vi "Determine Steps.vi"(8 "error in (no error)":errorcluster, 11 "DataProcessor in":refnum<class "DataProcessor.lvclass">) -> (0 "error out":errorcluster, 3 "DataProcessor out":refnum<class "DataProcessor.lvclass">)   [LabVIEW 2020, in "Volatus.lvlib" / "DataProcessor.lvclass"]
uses:
  DataProcessor.lvclass
  DataProcessor.lvclass/DataProcessor.ctl
  Task/Task.lvclass
  VolatusConfig/VolatusConfigElement/VolatusConfigElement.lvclass
  Processing Type.ctl
  Volatus.lvlib
  VolatusConfig/Task/Task.lvclass
  C:/dev/lv20CE/relink/lv-volatus/VolatusConfig/VolatusConfigElement/VolatusConfigElement.lvclass
  C:/dev/lv20CE/relink/lv-volatus/VolatusConfig/Task/Task.lvclass
  C:/dev/lv20CE/relink/lv-volatus/Volatus/DataHandlerTask/DataHandlerTask.lvclass
  C:/dev/lv20CE/relink/lv-volatus/Volatus/Task/Task.lvclass
  C:/Program Files (x86)/National Instruments/LabVIEW 2020/vi.lib/ActorFramework/Actor/Actor.lvclass
  C:/dev/lv20CE/relink/lv-volatus/Volatus/TaskStateHandler/TaskStateHandler.lvclass
  C:/dev/lv20CE/relink/lv-volatus/Volatus/VectoMessageHandler/VectoMessageHandler.lvclass
  C:/dev/lv20CE/relink/lv-volatus/Volatus/API Provider/API Provider.lvclass
  C:/dev/lv20CE/relink/lv-volatus/Volatus/DataHandler/DataHandler.lvclass
  C:/dev/lv20CE/relink/lv-volatus/Volatus/DataProcessor/DataProcessor.lvclass
  C:/dev/lv20CE/relink/lv-volatus/Volatus/Abortable/Abortable.lvclass
  C:/dev/lv20CE/relink/lv-volatus/Volatus/Reconfigurable/Reconfigurable.lvclass
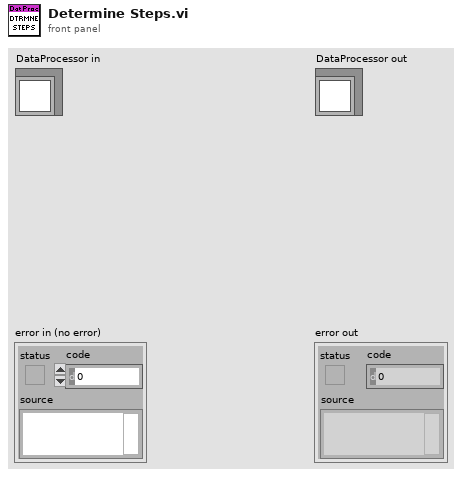
[diagram p1: front panel]
types:
  T1 = typedef "Volatus.lvlib/Processing Type.ctl" = enum16{"Scaling", "Redlines", "Logger"}
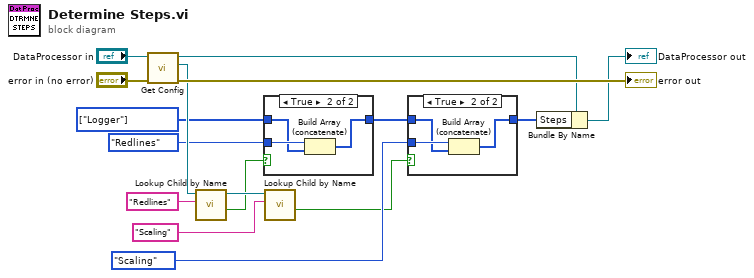
[diagram p0: block diagram]
diagram:
  w8 = T1[] [enum."Logger"] items=["Scaling", "Redlines", "Logger"] ("Array")
  n1 = call "Get Config.vi"("error in (no error)"="error in (no error)", "Task in"="DataProcessor in") -> ("error out"=→"error out":errorcluster, "Config"=w13:refnum<class "Task.lvclass">, "Task out"=w2:refnum<class "DataProcessor.lvclass">)  [unwired: 7 in]
  n2 = call "Lookup Child by Name.vi"("Child Name"="Redlines", "VolatusConfigElement in"=w13) -> ("Found"=w9:bool, "VolatusConfigElement out"=w10:refnum<class "Task.lvclass">)  [unwired: 6 in, 2 out]
  n3 = case shown="True" w9 {
    tunnel: w8 -> [w17 w19]
    tunnel: Processing_Type."Redlines" ("Processing Type") -> [_ w20]
    tunnel: [w17 w18] -> w6
    frame False {
    }
    frame True {
      n4 = Build Array (concatenate)(w20, w19) -> (w18:T1[])
    }
  }
  n5 = call "Lookup Child by Name.vi"("Child Name"="Scaling", "VolatusConfigElement in"=w10) -> ("Found"=w4:bool)  [unwired: 6 in, 3 out]
  n6 = case shown="True" w4 {
    tunnel: w6 -> [w21 w23]
    tunnel: Processing_Type."Scaling" ("Processing Type") -> [_ w24]
    tunnel: [w21 w22] -> w3
    frame False {
    }
    frame True {
      n7 = Build Array (concatenate)(w24, w23) -> (w22:T1[])
    }
  }
  n8 = Bundle By Name(cluster=w2, "Steps"=w3) -> (→"DataProcessor out":refnum<class "DataProcessor.lvclass">)
